vi "Lab 1.vi"() -> ()   [LabVIEW 2021]
panel:
  out "Thermometer":dbl(slide) scale=0.0..100.0
  in  "Celcius":dbl
  in  "To End:":bool
  out "Subtraction - Output":dbl
  out "Addition - Output":dbl
  in  "2nd Input":dbl
  in  "1st Input":dbl
  # "F = 1.8C + 32"
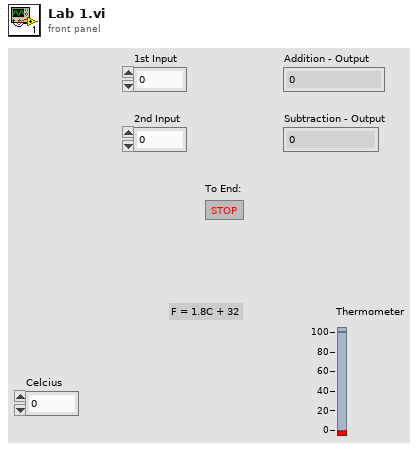
[diagram p1: front panel]
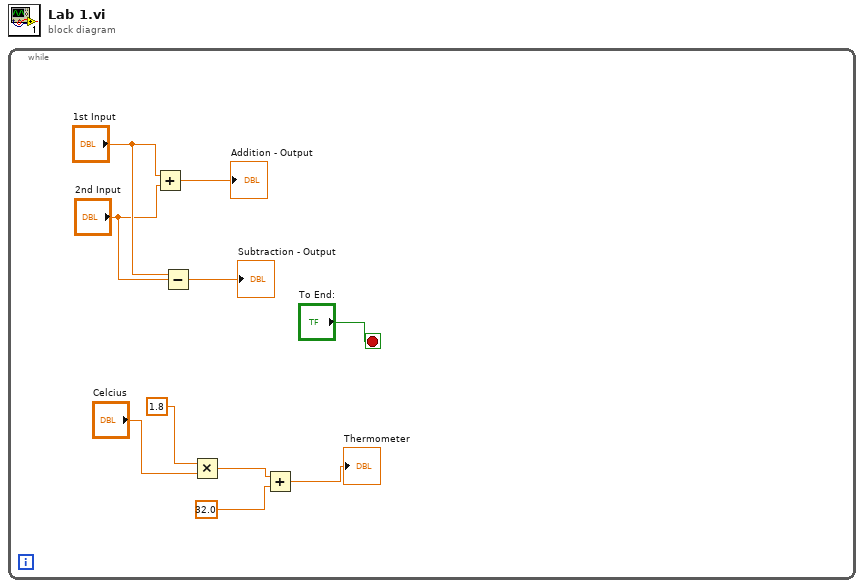
[diagram p0: block diagram]
diagram:
  n1 = while {
    stop <- "To End:" stop-if-true
    n2 = Add(x="1st Input", y="2nd Input") -> (x+y=→"Addition - Output":dbl)
    n3 = Subtract(x="1st Input", y="2nd Input") -> (x-y=→"Subtraction - Output":dbl)
    n4 = Multiply(x=1.8, y="Celcius") -> (x*y=w5:dbl)
    n5 = Add(x=w5, y=32.0) -> (x+y=→"Thermometer":dbl)
  }
